vi "USB Scan Device.vi"(11 "pDevNum":i32) -> (2 "function return":i32, 3 "pDevNum out":i32)   [LabVIEW 2010, in "usb_device.lvlib"]
doc: "int WINAPI USB_ScanDevice(int *pDevNum);"
uses:
  usb_device.lvlib
  USB2XXX.dll
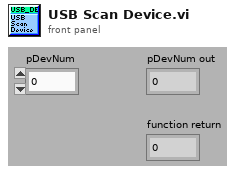
[diagram p1: front panel]
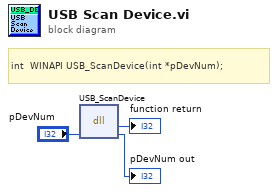
[diagram p0: block diagram]
diagram:
  # "int  WINAPI USB_ScanDevice(int *pDevNum);"
  n1 = dll-call lib="G:/OtherWork/USB2XXX_Example/trunk/Labview/PublicFiles/usb_device/USB2XXX.*" fn="USB_ScanDevice"("pDevNum"="pDevNum") -> (→"function return":i32, "pDevNum"=→"pDevNum out":i32)  [unwired: 3 in, 2 out]
